vi "Download_RunningStats.vi"(9 "Length":i64, 10 "Position":i64, 11 "DownloadStats In":T1) -> (3 "RunningStats":T1)   [LabVIEW 2018, in "HttpClient_NET.lvlib" / "HttpContent.lvclass"]
doc: "<b> </b> <b> </b>\nHttpClient_NET\nJustin Young - Viviota\nCopyright (c) 2021\nLicense: BSD"
uses:
  HttpContent.lvclass
  Types/DownloadStats_Cluster.ctl
  HttpClient_NET.lvlib
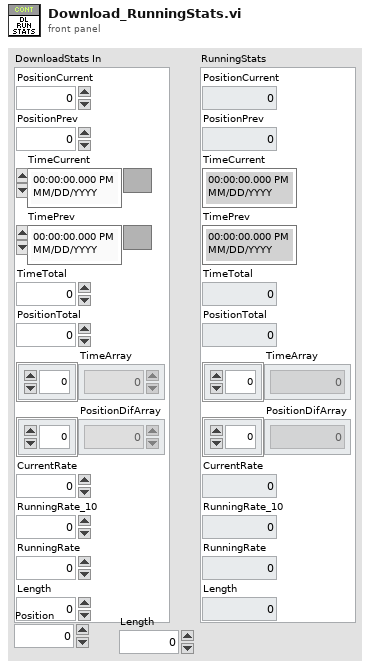
[diagram p1: front panel]
types:
  T1 = typedef "HttpClient_NET.lvlib/DownloadStats_Cluster.ctl" = cluster{"PositionCurrent":dbl, "PositionPrev":dbl, "TimeCurrent":timestamp, "TimePrev":timestamp, "TimeTotal":dbl, "PositionTotal":dbl, "TimeArray":dbl[], "PositionDifArray":dbl[], "CurrentRate":dbl, "RunningRate_10":dbl, "RunningRate":dbl, "Length":dbl}
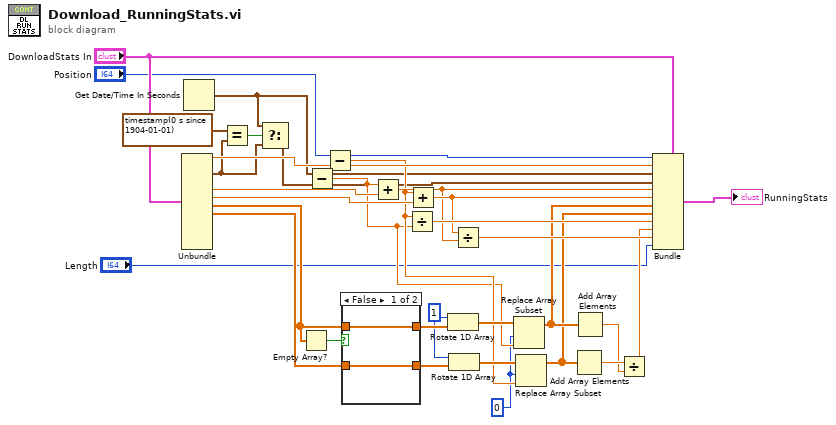
[diagram p0: block diagram]
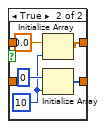
[diagram p2: hidden frame]
diagram:
  w12 = 0 ("index")
  w17 = 1 ("n")
  n1 = Unbundle("DownloadStats In") -> ("PositionCurrent"=w29:dbl, "TimeCurrent"=w2:timestamp, "TimeTotal"=w28:dbl, "PositionTotal"=w27:dbl, "TimeArray"=w21:dbl[], "PositionDifArray"=w20:dbl[])  [unwired: 6 out]
  n2 = Get Date/Time In Seconds() -> (seconds since 1Jan1904=w4:timestamp)
  n3 = Equal?(x=timestamp(0 s since 1904-01-01) ("TimePrev"), y=w2) -> (x = y?=w5:bool)
  n4 = Select(t=w4, s=w5, f=w2) -> (s? t:f=w3:timestamp)
  n5 = Empty Array?(array=w21) -> (empty?=w22:bool)
  n6 = Subtract(x=w4, y=w3) -> (x-y=w13:dbl)
  n7 = Subtract(x="Position", y=w29) -> (x-y=w14:dbl)
  n8 = case shown="False" w22 {
    tunnel: [w34 w36] -> w19
    tunnel: [w33 w35] -> w18
    tunnel: w21 -> [w34 _]
    tunnel: w20 -> [w33 _]
    frame False {
    }
    frame True {
      w37 = i64 10 ("PositionTotal")
      n9 = Initialize Array(0.0, w37) -> (w36:dbl[])
      n10 = Initialize Array(i64 0 ("PositionTotal"), w37) -> (w35:i64[])
    }
  }
  n11 = Add(x=w13, y=w28) -> (x+y=w24:dbl)
  n12 = Divide(x=w14, y=w13) -> (x/y=w26:dbl)
  n13 = Add(x=w14, y=w27) -> (x+y=w25:dbl)
  n14 = Rotate 1D Array(1:w19, 2:w17) -> (0:w16:dbl[])
  n15 = Rotate 1D Array(1:w18, 2:w17) -> (0:w15:dbl[])
  n16 = Divide(x=w25, y=w24) -> (x/y=w23:dbl)
  n17 = Replace Array Subset(array=w16, new element=w13, index=w12) -> (w11:dbl[])
  n18 = Replace Array Subset(array=w15, new element=w14, index=w12) -> (w10:dbl[])
  n19 = Add Array Elements(numeric array=w10) -> (sum=w9:dbl)
  n20 = Add Array Elements(numeric array=w11) -> (sum=w8:dbl)
  n21 = Divide(x=w9, y=w8) -> (x/y=w7:dbl)
  n22 = Bundle(cluster="DownloadStats In", "PositionCurrent"="Position", "PositionPrev"=w29, "TimeCurrent"=w4, "TimePrev"=w3, "TimeTotal"=w24, "PositionTotal"=w25, "TimeArray"=w11, "PositionDifArray"=w10, "CurrentRate"=w26, "RunningRate_10"=w7, "RunningRate"=w23, "Length"="Length") -> (→"RunningStats":T1)
